vi "AMZ_S3_APIHLP_Convert Versioning Status to Enum.vi"(4 "Status String":string) -> (1 "Status":T1)   [LabVIEW 2015, in "LV Interface for Amazon S3.lvlib"]
doc: "Convert the Storage Class represented as a String to the Enum typedef representation."
uses:
  LV Interface for Amazon S3.lvlib
  Typedefs/AMZ_S3_Versioning Status.ctl
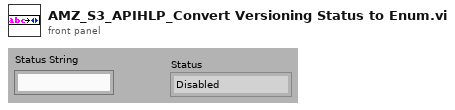
[diagram p1: front panel]
types:
  T1 = typedef "LV Interface for Amazon S3.lvlib/AMZ_S3_Versioning Status.ctl" = enum16{"Disabled", "Suspended", "Enabled"}
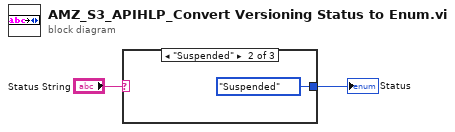
[diagram p0: block diagram]
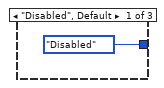
[diagram p2: hidden frame]
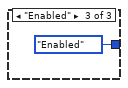
[diagram p3: hidden frame]
diagram:
  n1 = case shown="\"Suspended\"" "Status String" {
    tunnel: [AMZ_S3_Versioning_Status."Disabled" ("Status") AMZ_S3_Versioning_Status."Suspended" ("Status") AMZ_S3_Versioning_Status."Enabled" ("Status")] -> w1
    frame "Disabled", Default {
    }
    frame "Suspended" {
    }
    frame "Enabled" {
    }
  }
  "Status" <- w1
